vi "RTS Date Time.vi"() -> ()   [LabVIEW 2016]
uses:
  <vilib>/Utility/miscctls.llb/LVDateTimeRec.ctl
panel:
  out "Numeric 2":dbl format="%#_6f"
  in  "Numeric":dbl format="%<%H:%M:%S>T"
  out "s? t:f":i32
  out "Timestamp from Date/Time String":timestamp
  out "Current Timestamp":timestamp
  out "Number of Seconds":dbl
  out "Timestamp from Number of Seconds":timestamp
  out "Sample Date String Input":string
  out "Sample Time String Input":string
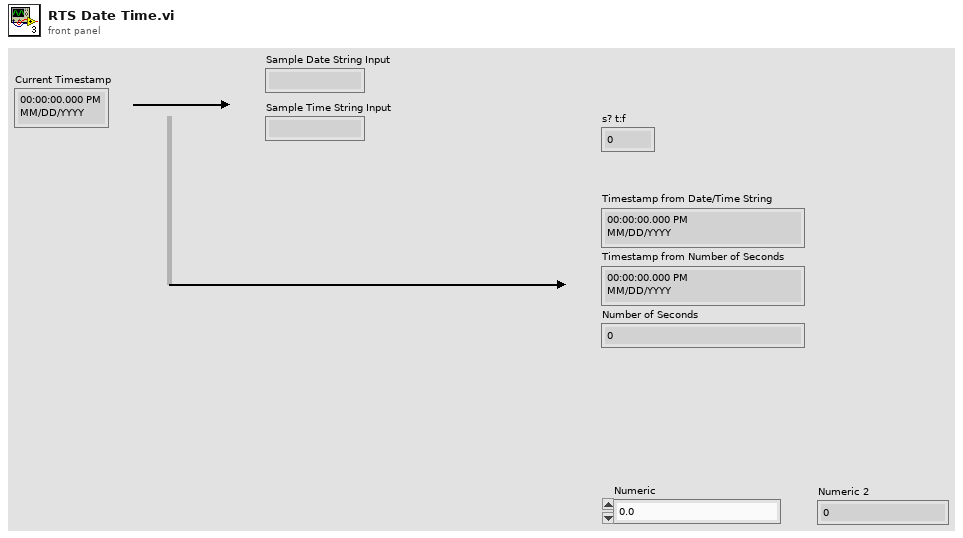
[diagram p1: front panel]
types:
  T1 = typedef "LVDateTimeRec.ctl" = cluster{"fractional second":dbl, "second":i32, "minute":i32, "hour":i32, "day of month":i32, "month":i32, "year":i32, "day of week":i32, "day of year":i32, "DST":i32}
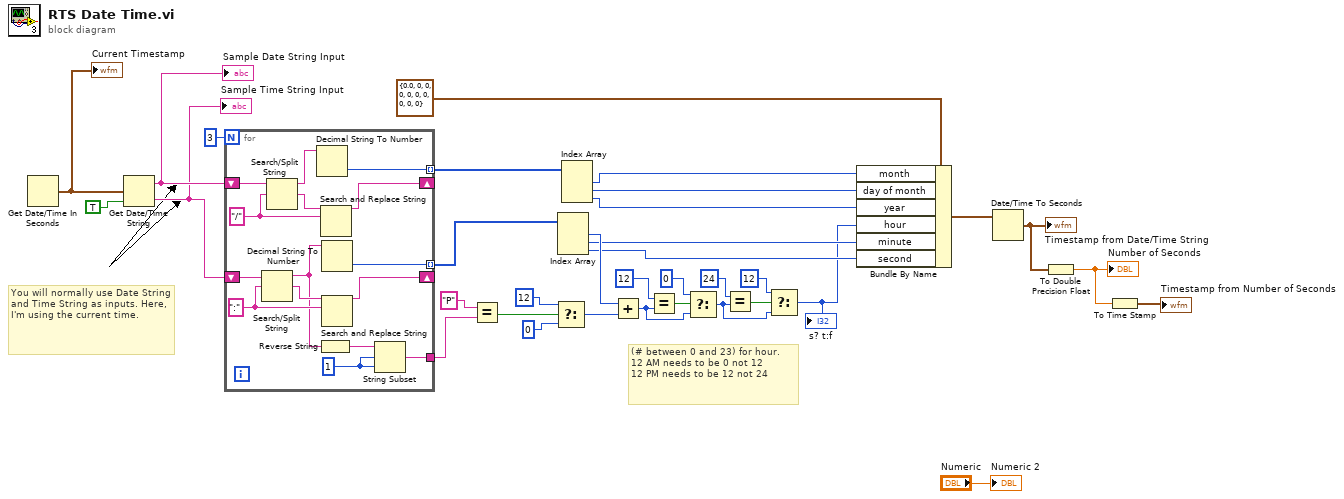
[diagram p0: block diagram]
diagram:
  # "You will normally use Date String and Time String as inputs. Here, I'm using the current time."
  # "(# between 0 and 23) for hour.\n12 AM needs to be 0 not 12\n12 PM needs to be 12 not 24"
  n1 = Get Date/Time In Seconds() -> (seconds since 1Jan1904=w34:timestamp)
  "Current Timestamp" <- w34
  n2 = Get Date/Time String(seconds (now)=w34, want seconds? (F)=TRUE) -> (date string=w31:string, time string=w30:string)  [unwired: 1 in]
  "Sample Date String Input" <- w31
  "Sample Time String Input" <- w30
  n3 = for {
    N: 3 -> [_]
    shift-right: [w47] -> _
    shift-left: w31 -> [w48]
    tunnel: [w45] -> w20 mode=indexing
    shift-right: [w44] -> _
    shift-left: w30 -> [w40]
    tunnel: [w41] -> w27 mode=indexing
    tunnel: [w35] -> w29
    w36 = 1 ("offset (0)")
    w42 = ":" ("search string/char (-)")
    w43 = "/" ("search string/char (-)")
    n4 = Search/Split String(string=w40, search string/char (-)=w42) -> (substring before match=w38:string, match + rest of string=w39:string)  [unwired: 1 in, 1 out]
    n5 = Search/Split String(string=w48, search string/char (-)=w43) -> (substring before match=w46:string, match + rest of string=w49:string)  [unwired: 1 in, 1 out]
    n6 = Decimal String To Number(string=w46) -> (number=w45:i32)  [unwired: 2 in, 1 out]
    n7 = Reverse String(1:w38) -> (0:w37:string)
    n8 = Search and Replace String(input string=w49, search string=w43) -> (result string=w47:string)  [unwired: 6 in, 3 out]
    n9 = Decimal String To Number(string=w38) -> (number=w41:i32)  [unwired: 2 in, 1 out]
    n10 = Search and Replace String(input string=w39, search string=w42) -> (result string=w44:string)  [unwired: 6 in, 3 out]
    n11 = String Subset(string=w37, offset (0)=w36, length (rest)=w36) -> (substring=w35:string)
  }
  n12 = Equal?(x="P", y=w29) -> (x = y?=w26:bool)
  n13 = Select(t=12 ("index"), s=w26, f=0 ("index")) -> (s? t:f=w23:i32)
  n14 = Index Array(array=w27) -> (element #1=w22:i32, element #2=w16:i32, element #3=w15:i32)  [unwired: 3 in]
  n15 = Index Array(array=w20) -> (element #1=w19:i32, element #2=w18:i32, element #3=w17:i32)  [unwired: 3 in]
  n16 = Add(x=w22, y=w23) -> (x+y=w9:i32)
  n17 = Equal?(x=12 ("y"), y=w9) -> (x = y?=w11:bool)
  n18 = Select(t=0, s=w11, f=w9) -> (s? t:f=w6:i32)
  n19 = Equal?(x=24 ("y"), y=w6) -> (x = y?=w13:bool)
  n20 = Select(t=12 ("index"), s=w13, f=w6) -> (s? t:f=w5:i32)
  "s? t:f" <- w5
  n21 = Bundle By Name(cluster=T1 {"fractional second"=0.0, "second"=0, "minute"=0, "hour"=0, "day of month"=0, "month"=0, "year"=0, "day of week"=0, "day of year"=0, "DST"=0} ("date time rec"), "month"=w19, "day of month"=w18, "year"=w17, "hour"=w5, "minute"=w16, "second"=w15) -> (w14:T1)
  n22 = Date/Time To Seconds(2:w14) -> (0:w4:timestamp)  [unwired: 1 in]
  "Timestamp from Date/Time String" <- w4
  n23 = To Double Precision Float(number=w4) -> (double precision float=w3:dbl)
  "Number of Seconds" <- w3
  n24 = To Time Stamp(1:w3) -> (0:→"Timestamp from Number of Seconds":timestamp)
  "Numeric 2" <- "Numeric"
